vi "Interpolate Lift System.vi"(8 "Duration":dbl, 9 "Current Time":dbl, 10 "End Lift System Actions":T1, 11 "Start Lift System Actions":T1) -> (3 "Current Lift System Actions":T1)   [LabVIEW 2019]
uses:
  Controls/Lift System Actions.ctl
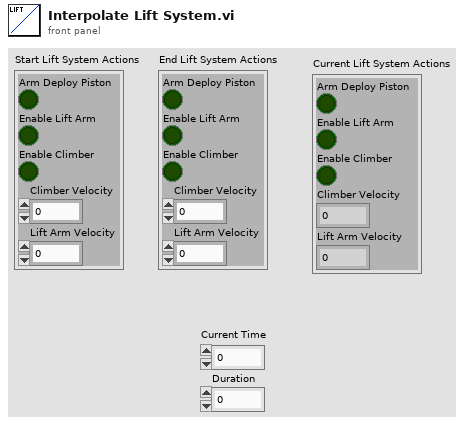
[diagram p1: front panel]
types:
  T1 = typedef "Lift System Actions.ctl" = cluster{"Arm Deploy Piston":bool, "Enable Lift Arm":bool, "Enable Climber":bool, "Climber Velocity":dbl, "Lift Arm Velocity":dbl}
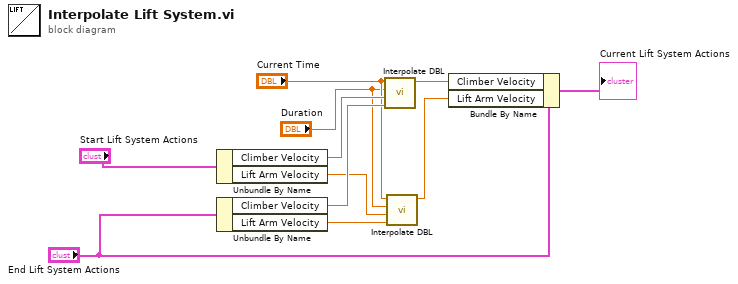
[diagram p0: block diagram]
diagram:
  n1 = Unbundle By Name("Start Lift System Actions") -> ("Climber Velocity"=w11:dbl, "Lift Arm Velocity"=w2:dbl)
  n2 = Unbundle By Name("End Lift System Actions") -> ("Climber Velocity"=w10:dbl, "Lift Arm Velocity"=w1:dbl)
  n3 = call "Interpolate DBL.vi"("Ending Value"=w10, "Starting Value"=w11, "Duration"="Duration", "Current Time"="Current Time") -> ("Current Value"=w9:dbl)  [unwired: 7 in]
  n4 = call "Interpolate DBL.vi"("Ending Value"=w1, "Starting Value"=w2, "Duration"="Duration", "Current Time"="Current Time") -> ("Current Value"=w5:dbl)  [unwired: 7 in]
  n5 = Bundle By Name(cluster="End Lift System Actions", "Climber Velocity"=w9, "Lift Arm Velocity"=w5) -> (→"Current Lift System Actions":T1)
